vi "VacuumSwitchTest.vi"(3 "Error In":errorcluster, 5 "ControlType":T1(ring)=enum."DecimalSwitch", 6 "DecimalIn":u32) -> (0 "error out":errorcluster, 1 "DecimalOut":u32, 2 "data":bool[](array[boolean]) caption="Sensor status")   [LabVIEW 2019]
panel:
  in  "8.GantryHead":cluster{"GH5":bool, "GH6":bool}
  in  "7.No connection":cluster{"NC1":bool, "NC2":bool}
  in  "6.GantryHead":T2
  in  "5.SensorPCBTray":cluster{"ST1":bool, "ST2":bool, "ST3":bool}
  in  "4.Sensor/PCB":T3
  in  "3.PickupTool":T4
  in  "2.BasePlateTray":cluster{"BPT1":bool, "BPT2":bool, "BPT3":bool}
  in  "1.BasePlate":T5
  out "DecimalExpected":u32
  # "2.BPT1"
  # "2.BPT3"
  # "2.BPT2"
  # "1.BP1"
  # "1.BP6"
  # "6.Plate"
  # "6.Tool"
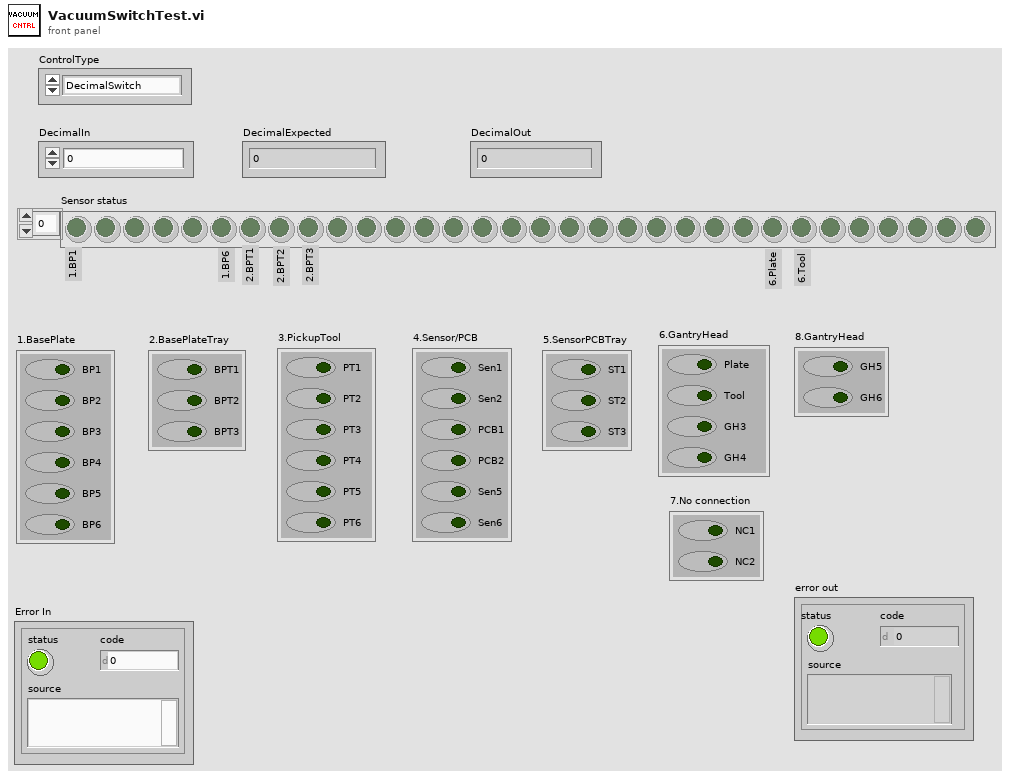
[diagram p1: front panel]
types:
  T1 = enum16{"Conversion", "BinarySwitch", "DecimalSwitch"}
  T2 = cluster{"Plate":bool, "Tool":bool, "GH3":bool, "GH4":bool}
  T3 = cluster{"Sen1":bool, "Sen2":bool, "PCB1":bool, "PCB2":bool, "Sen5":bool, "Sen6":bool}
  T4 = cluster{"PT1":bool, "PT2":bool, "PT3":bool, "PT4":bool, "PT5":bool, "PT6":bool}
  T5 = cluster{"BP1":bool, "BP2":bool, "BP3":bool, "BP4":bool, "BP5":bool, "BP6":bool}
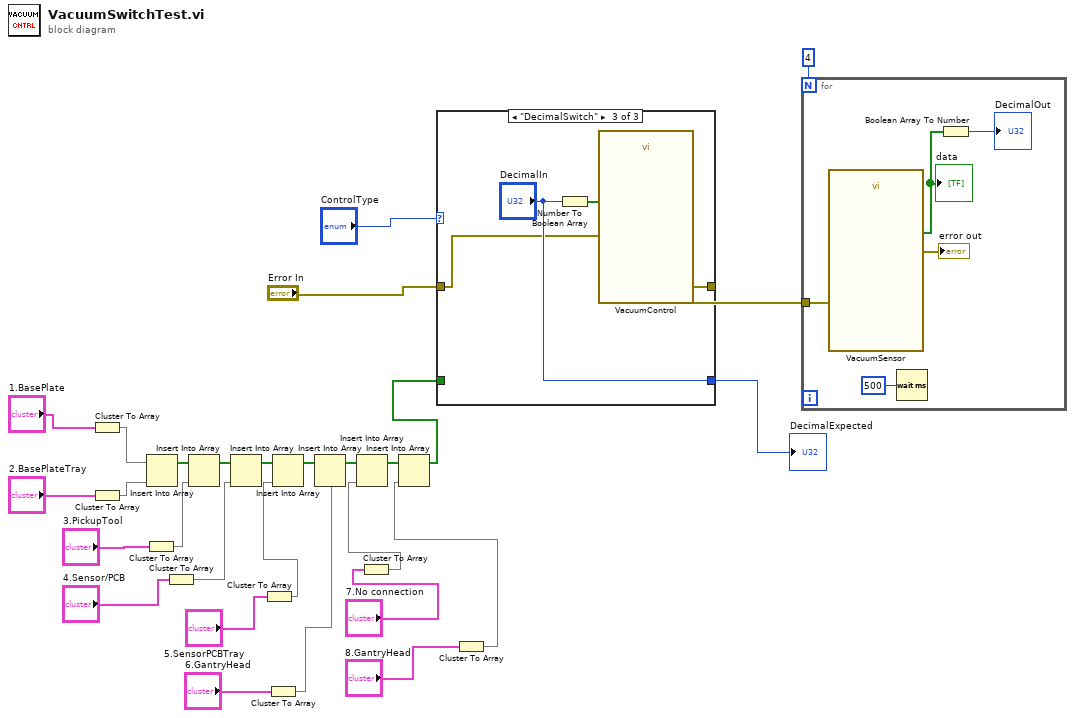
[diagram p0: block diagram]
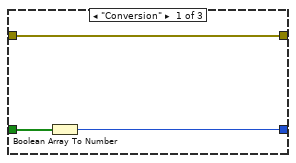
[diagram p2: hidden frame]
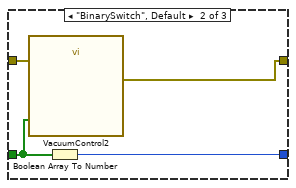
[diagram p3: hidden frame]
diagram:
  n1 = Cluster To Array(cluster="1.BasePlate") -> (array=w20:bool[])
  n2 = Cluster To Array(cluster="2.BasePlateTray") -> (array=w19:bool[])
  n3 = Cluster To Array(cluster="3.PickupTool") -> (array=w17:bool[])
  n4 = Insert Into Array(array=w20, new element=w19) -> (w18:bool[])  [unwired: 1 in]
  n5 = Cluster To Array(cluster="4.Sensor/PCB") -> (array=w15:bool[])
  n6 = Insert Into Array(array=w18, new element=w17) -> (w16:bool[])  [unwired: 1 in]
  n7 = Insert Into Array(array=w16, new element=w15) -> (w14:bool[])  [unwired: 1 in]
  n8 = Cluster To Array(cluster="5.SensorPCBTray") -> (array=w13:bool[])
  n9 = Cluster To Array(cluster="6.GantryHead") -> (array=w11:bool[])
  n10 = Insert Into Array(array=w14, new element=w13) -> (w12:bool[])  [unwired: 1 in]
  n11 = Insert Into Array(array=w12, new element=w11) -> (w10:bool[])  [unwired: 1 in]
  n12 = Cluster To Array(cluster="7.No connection") -> (array=w9:bool[])
  n13 = Insert Into Array(array=w10, new element=w9) -> (w8:bool[])  [unwired: 1 in]
  n14 = Cluster To Array(cluster="8.GantryHead") -> (array=w7:bool[])
  n15 = Insert Into Array(array=w8, new element=w7) -> (w6:bool[])  [unwired: 1 in]
  n16 = case shown="\"DecimalSwitch\"" "ControlType" {
    tunnel: w6 -> [w31 w34 _]
    tunnel: [w30 w35 "DecimalIn"] -> w5
    tunnel: "Error In" -> [w29 w33 w37]
    tunnel: [w29 w32 w36] -> w2
    frame "Conversion" {
      n17 = Boolean Array To Number(Boolean array=w31) -> (number=w30:u32)
    }
    frame "BinarySwitch", Default {
      n18 = call "VacuumControl2"("data"=w34, "error in"=w33) -> ("error out"=w32:errorcluster)  [unwired: 16 in, 1 out]
      n19 = Boolean Array To Number(Boolean array=w34) -> (number=w35:u32)
    }
    frame "DecimalSwitch" {
      n20 = Number To Boolean Array(number="DecimalIn") -> (Boolean array=w39:bool[])
      n21 = call "VacuumControl"("data"=w39, "error in"=w37) -> ("error out"=w36:errorcluster)  [unwired: 16 in, 1 out]
    }
  }
  "DecimalExpected" <- w5
  n22 = for {
    N: 4 -> [_]
    tunnel: w2 -> [w41]
    n23 = call "VacuumSensor"("error in"=w41) -> ("data"=w43:bool[], "error out"=→"error out":errorcluster)  [unwired: 16 in, 1 out]
    "data" <- w43
    n24 = Wait (ms)(milliseconds to wait=u32 500) -> ()  [unwired: 1 out]
    n25 = Boolean Array To Number(Boolean array=w43) -> (number=→"DecimalOut":u32)
  }
